vi "Configure Trigger Source [TRG] Core.vi"(8 "error in (no error)":errorcluster, 9 "source (Immediate)":i32(ring) items=["Immediate", "External", "Software", "TTL0", "TTL1", "TTL2", "TTL3", "TTL4", "TTL5", "TTL6", "TTL7", "ECL0", "ECL1", "PXI Star", "RTSI 0", "RTSI 1", "RTSI 2", "RTSI 3", "RTSI 4", "RTSI 5", "RTSI 6"], 10 "channel name (\"CHANNEL1\")":string="CHANNEL1", 11 "CS++DCPwr in":refnum<class "CS++DCPwr.lvclass">) -> (0 "error out":errorcluster, 3 "CS++DCPwr out":refnum<class "CS++DCPwr.lvclass">)   [LabVIEW 2013, in "CS++DCPwr.lvlib" / "CS++DCPwr.lvclass"]
doc: "This VI configures the trigger source to which the power supply responds after you call IviDCPwr Initiate [TRG]. When the power supply receives a trigger signal on the source you specify, it changes its current and voltage outputs.\n\nYou configure the triggered current and voltage outputs with the\nIviDCPwr Configure Triggered Current Limit [TRG] and \nIviDCPwr Configure Triggered Voltage Level [TRG] VIs. \n\nNotes:\n\n(1) This VI is part of the IviDCPwrTrigger [TRG] extension group."
uses:
  CS++DCPwr.lvclass
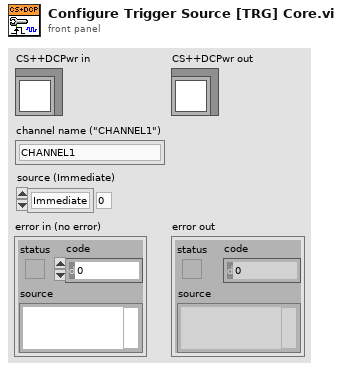
[diagram p1: front panel]
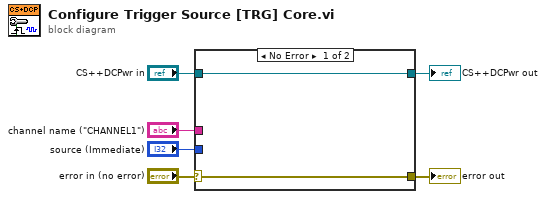
[diagram p0: block diagram]
diagram:
  n1 = case shown="No Error" "error in (no error)" {
    selector: "error in (no error)" -> [w7 w10]
    tunnel: [w7 w10] -> w5
    tunnel: [w8 w9] -> w3
    tunnel: "CS++DCPwr in" -> [w8 w9]
    tunnel: "channel name (\"CHANNEL1\")" -> [_ _]
    tunnel: "source (Immediate)" -> [_ _]
    frame No Error {
    }
    frame Error {
    }
  }
  "error out" <- w5
  "CS++DCPwr out" <- w3
